vi "Update Status Log.vi"(10 "Status in":string, 11 "Status Array":string[](array[string])) -> (2 "Status out":string, 3 "Status out":string[](array[string]))   [LabVIEW 2020, in "Dashboard.lvlib"]
uses:
  Dashboard.lvlib
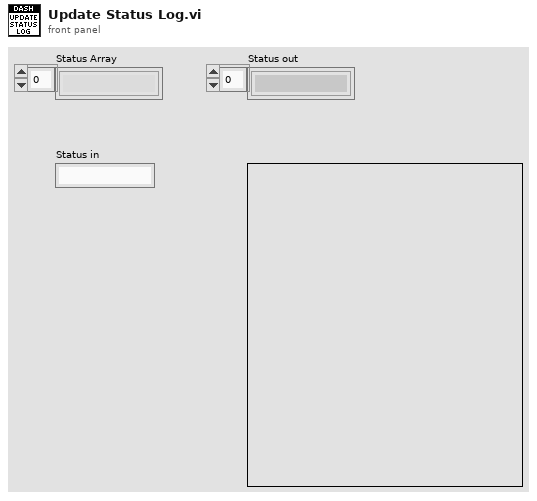
[diagram p1: front panel]
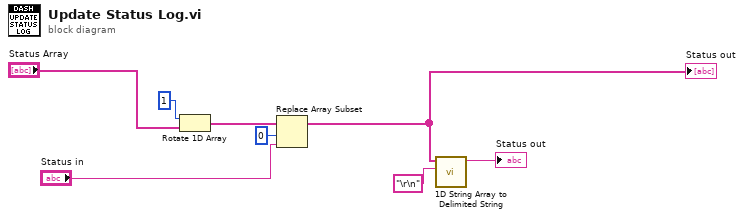
[diagram p0: block diagram]
diagram:
  n1 = Rotate 1D Array(1:"Status Array", 2:1 ("n")) -> (0:w3:string[])
  n2 = Replace Array Subset(array=w3, new element="Status in", index=0) -> (w5:string[])
  "Status out" <- w5
  n3 = call <vilib>:"1D String Array to Delimited String.vi"("delimiter"="\r\n", "string array"=w5) -> ("delimited string"=→"Status out":string)  [unwired: 9 in]
